vi "Periodic Tasks.vi"(8 "error in":errorcluster) -> ()   [LabVIEW 2018]
doc: "This VI runs in parallel to other tasks. It can contain as many user-defined periodic loops as you need. These can carry out PID or other sorts of timed response."
uses:
  <vilib>/Rock Robotics/WPI/Solenoid/WPI_SolenoidValue.ctl
  <vilib>/Rock Robotics/Network Tables/NT Read Number.vi
  Globals.vi
  <vilib>/Rock Robotics/Network Tables/NT Write String.vi
  <vilib>/Rock Robotics/WPI/Solenoid/WPI_SolenoidSetEnum.vi
  navx-mxp/labview/navX Library v2/navX Library v2.lvlib
panel:
  out "navX axes":T1
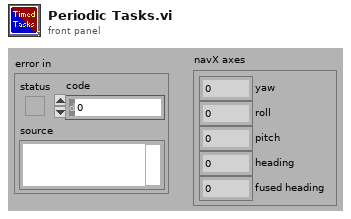
[diagram p1: front panel]
types:
  T1 = cluster{"yaw":dbl, "roll":dbl, "pitch":dbl, "heading":dbl, "fused heading":dbl}
  T2 = typedef "navX Library v2.lvlib/Z900_navX_DeviceTypeDef.ctl" = cluster{"Interface":cluster{"Protocol":T3, "Update Rate (4Hz-100Hz)":u8, "navX Open TypeDef":variant}, "Notify Packet":refnum<notifier>, "Loop VI Refnum":refnum<vi>, "Ready to Close Occurrence Refnum":refnum<k4>}
  T3 = typedef "navX Library v2.lvlib/Z900_navX_ProtocolTypeDef.ctl" = enum16{"SERIAL", "I2C", "SPI"}
  T4 = typedef "WPI_AnalogChannelDevRef.ctl" = cluster{"DevStatus":errorcluster, "Analog Channel":T5}
  T5 = typedef "FPGA_AIChannel.ctl" = enum8{"AI 0", "AI 1", "AI 2", "AI 3", "AI MXP 0", "AI MXP 1", "AI MXP 2", "AI MXP 3", "Invalid"}
  T6 = typedef "WPI_MotorControlDeviceRef.ctl" = cluster{"DeviceStatus":errorcluster, "Type":T7, "PWM":cluster{"PWM Channel":T8, "DeadBand":T9}, "CAN":cluster{"Device Number":u8, "SetOutput VI Ref":variant, "GetOutput VI Ref":variant, "Enable VI Ref":variant, "Disable VI Ref":variant, "Data":variant}, "Invert":bool, "DIO PWM":cluster{"PWM \"Enable\" Channel":T8, "DIOChannel":T10, "PWM Rate":dbl}}
  T7 = typedef "WPI_MotorControlType.ctl" = enum16{"PWM", "CAN", "DIO PWM"}
  T8 = typedef "FPGA_DIOPWMChannel.ctl" = enum8{"PWM 0", "PWM 1", "PWM 2", "PWM 3", "PWM 4", "PWM 5", "PWM 6", "PWM 7", "PWM 8", "PWM 9", "PWM MXP 0", "PWM MXP 1", "PWM MXP 2", "PWM MXP 3", "PWM MXP 4", "PWM MXP 5", "PWM MXP 6", "PWM MXP 7", "PWM MXP 8", "PWM MXP 9", "Invalid"}
  T9 = typedef "WPI_PWMDeadband.ctl" = cluster{"Name":string, "maxPositivePwm":i32, "minPositivePwm":i32, "centerPwm":i32, "maxNegativePwm":i32, "minNegativePwm":i32, "angularRange":u16}
  T10 = typedef "FPGA_DIOChannel.ctl" = enum8{"DIO 0", "DIO 1", "DIO 2", "DIO 3", "DIO 4", "DIO 5", "DIO 6", "DIO 7", "DIO 8", "DIO 9", "DIO MXP 0", "DIO MXP 1", "DIO MXP 2", "DIO MXP 3", "DIO MXP 4", "DIO MXP 5", "DIO MXP 6", "DIO MXP 7", "DIO MXP 8", "DIO MXP 9", "DIO MXP 10", "DIO MXP 11", "DIO MXP 12", "DIO MXP 13", "DIO MXP 14", "DIO MXP 15", "SPI Port CS1", "SPI Port CS2", "SPI Port CS3", "SPI Port MISO", "SPI Port MOSI", "Invalid"}
  T11 = typedef "WPI_EncoderDevRef.ctl" = cluster{"DevStatus":errorcluster, "EncoderIndex":T12, "CounterIndex":T13, "DistancePerCount":dbl, "Decoding Type":T14}
  T12 = typedef "FPGA_EncoderIdx.ctl" = enum8{"Enc 0", "Enc 1", "Enc 2", "Enc 3", "Enc 4", "Enc 5", "Enc 6", "Enc 7", "Invalid"}
  T13 = typedef "FPGA_CounterCtrSystemIndex.ctl" = enum8{"Ctr 0", "Ctr 1", "Ctr 2", "Ctr 3", "Ctr 4", "Ctr 5", "Ctr 6", "Ctr 7", "Invalid"}
  T14 = typedef "WPI_EncoderType.ctl" = enum16{"1x", "2x", "4x"}
  T15 = typedef "WPI_SolenoidDevRef.ctl" = cluster{"DevStatus":errorcluster, "Pneumatics Control Module":u8, "Forward Solenoid Channel":T16, "Reverse Solenoid Channel":T16}
  T16 = typedef "WPI_SolenoidChannel.ctl" = enum8{"Solenoid 0", "Solenoid 1", "Solenoid 2", "Solenoid 3", "Solenoid 4", "Solenoid 5", "Solenoid 6", "Solenoid 7", "Invalid"}
  T17 = typedef "WPI_SolenoidValue.ctl" = enum16{"Off", "On", "Forward", "Reverse"}
  T18 = cluster{"Yaw":dbl, "Roll":dbl, "Pitch":dbl, "Heading":dbl, "Fused Heading":dbl}
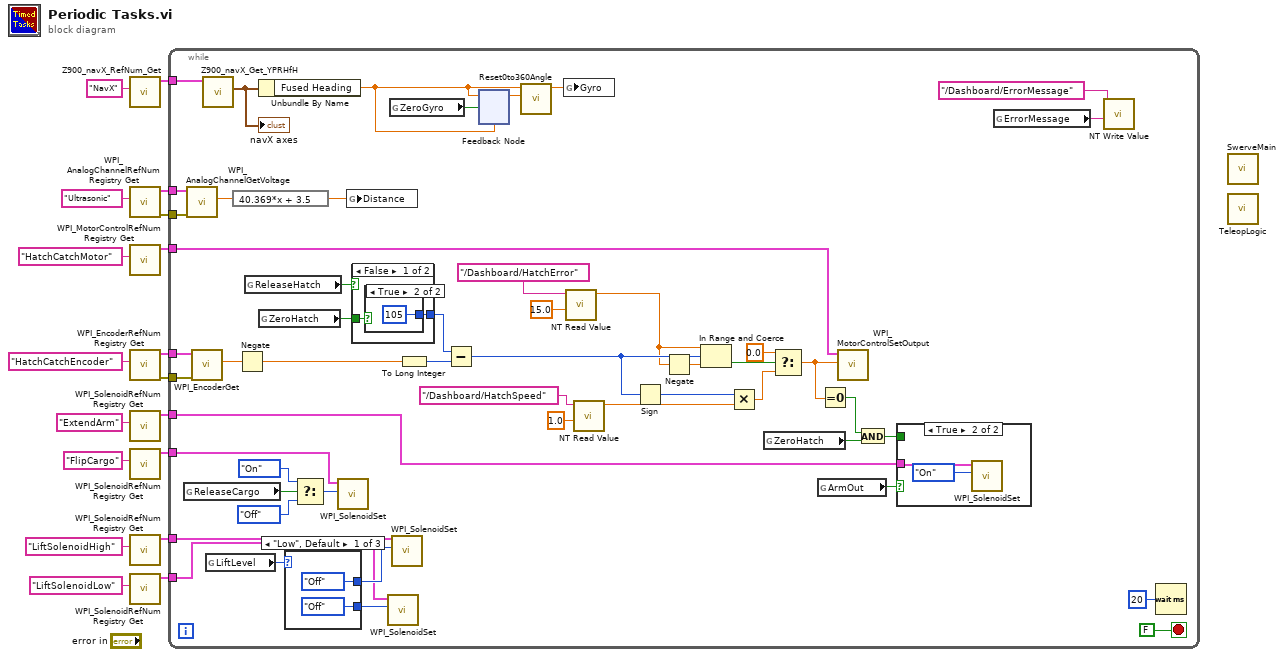
[diagram p0: block diagram]
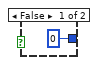
[diagram p3: hidden frame]
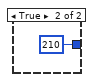
[diagram p4: hidden frame]
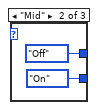
[diagram p5: hidden frame]
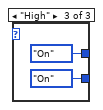
[diagram p6: hidden frame]
diagram:
  n1 = call "Z900_navX_RefNum_Get.vi"("refnum name"="NavX") -> ("navX Device"=w17:T2)  [unwired: 9 in, 1 out]
  n2 = call <vilib>:"WPI_AnalogChannelRefNum Registry Get.vi"("refnum name"="Ultrasonic") -> ("error out"=w15:errorcluster, "AIDeviceRef"=w2:T4)  [unwired: 9 in]
  n3 = call <vilib>:"WPI_MotorControlRefNum Registry Get.vi"("refnum name"="HatchCatchMotor") -> ("MotorControlDevRef"=w14:T6)  [unwired: 9 in, 1 out]
  n4 = call <vilib>:"WPI_EncoderRefNum Registry Get.vi"("refnum name"="HatchCatchEncoder") -> ("error out"=w6:errorcluster, "EncoderDevRef"=w7:T11)  [unwired: 9 in]
  n5 = call <vilib>:"WPI_SolenoidRefNum Registry Get.vi"("refnum name"="ExtendArm") -> ("SolenoidDevRef"=w1:T15)  [unwired: 9 in, 1 out]
  n6 = call <vilib>:"WPI_SolenoidRefNum Registry Get.vi"("refnum name"="FlipCargo") -> ("SolenoidDevRef"=w3:T15)  [unwired: 9 in, 1 out]
  n7 = call <vilib>:"WPI_SolenoidRefNum Registry Get.vi"("refnum name"="LiftSolenoidHigh") -> ("SolenoidDevRef"=w13:T15)  [unwired: 9 in, 1 out]
  n8 = call <vilib>:"WPI_SolenoidRefNum Registry Get.vi"("refnum name"="LiftSolenoidLow") -> ("SolenoidDevRef"=w12:T15)  [unwired: 9 in, 1 out]
  n9 = while {
    tunnel: w17 -> [w42]
    tunnel: w2 -> [w64]
    tunnel: w15 -> [w63]
    tunnel: w14 -> [w33]
    tunnel: w13 -> [w58]
    tunnel: w12 -> [w59]
    tunnel: w7 -> [w57]
    tunnel: w6 -> [w56]
    tunnel: w3 -> [w49]
    tunnel: w1 -> [w21]
    stop <- FALSE stop-if-true
    n10 = global read "Globals.vi" "ReleaseCargo"() -> (w53:bool)
    n11 = call <vilib>:"WPI_AnalogChannelGetVoltage.vi"("error in (no error)"=w63, "AIDeviceRef"=w64) -> ("Voltage"=w32:dbl)  [unwired: 7 in, 2 out]
    n12 = call <vilib>:"WPI_EncoderGet.vi"("error in (no error)"=w56, "EncoderDevRef"=w57) -> ("Distance"=w23:dbl)  [unwired: 4 in, 5 out]
    n13 = call "Z900_navX_Get_YPRHfH.vi"("navX Device"=w42) -> ("YRPHfH"=w67:T18)  [unwired: 7 in, 3 out]
    "navX axes" <- w67
    n14 = global read "Globals.vi" "LiftLevel"() -> (w62:enum16{"Low", "Mid", "High"})
    n15 = expression code="40.369*x + 3.5"(w32) -> (w31:dbl)
    n16 = Negate(x=w23) -> (-x=w22:dbl)
    n17 = global read "Globals.vi" "ReleaseHatch"() -> (w47:bool)
    n18 = Unbundle By Name(w67) -> ("Fused Heading"=w48:dbl)
    n19 = global read "Globals.vi" "ZeroHatch"() -> (w19:bool)
    n20 = case shown="\"Low\", Default" w62 {
      tunnel: [WPI_SolenoidValue."Off" ("Value") WPI_SolenoidValue."Off" ("Value") WPI_SolenoidValue."On" ("Value")] -> w61
      tunnel: [WPI_SolenoidValue."Off" ("Value") WPI_SolenoidValue."On" ("Value") WPI_SolenoidValue."On" ("Value")] -> w60
      frame "Low", Default {
      }
      frame "Mid" {
      }
      frame "High" {
      }
    }
    n21 = Select(t=WPI_SolenoidValue."On" ("Value"), s=w53, f=WPI_SolenoidValue."Off") -> (s? t:f=w50:T17)
    n22 = call-poly <vilib>:"WPI_SolenoidSet.vi"("Value"=w50, "SolenoidDevRef"=w49) -> ()  [unwired: 8 in, 2 out]
    n23 = global write "Globals.vi" "Distance"(w31) -> ()
    n24 = case shown="False" w47 {
      tunnel: w19 -> [w73 _]
      tunnel: [w72 210] -> w24
      frame False {
        n25 = case shown="True" w73 {
          tunnel: [0 105] -> w72
          frame False {
          }
          frame True {
          }
        }
      }
      frame True {
      }
    }
    n26 = call-poly <vilib>:"WPI_SolenoidSet.vi"("Value"=w60, "SolenoidDevRef"=w59) -> ()  [unwired: 8 in, 2 out]
    n27 = global read "Globals.vi" "ZeroGyro"() -> (w65:bool)
    n28 = call-poly <vilib>:"WPI_SolenoidSet.vi"("Value"=w61, "SolenoidDevRef"=w58) -> ()  [unwired: 8 in, 2 out]
    n29 = To Long Integer(number=w22) -> (32bit integer=w46:i32)
    n30 = Subtract(x=w24, y=w46) -> (x-y=w43:i32)
    n31 = feedback-in #1(w48, w65) -> ()
    n32 = feedback #1(w48) -> (w68:dbl)
    n33 = call "Reset0to360Angle.vi"("Offset"=w68, "AngleInput"=w48) -> ("AngleOutput"=w66:dbl)  [unwired: 9 in]
    n34 = global write "Globals.vi" "Gyro"(w66) -> ()
    n35 = call-poly <vilib>:"NT Read Value.vi"("Default Value"=15.0, "Name"="/Dashboard/HatchError") -> ("Numeric"=w25:dbl)  [unwired: 8 in, 1 out]
    n36 = call-poly <vilib>:"NT Read Value.vi"("Default Value"=1.0, "Name"="/Dashboard/HatchSpeed") -> ("Numeric"=w28:dbl)  [unwired: 8 in, 1 out]
    n37 = Sign(1:w43) -> (0:w44:i32)
    n38 = Negate(x=w25) -> (-x=w36:dbl)
    n39 = In Range and Coerce(upper limit=w25, x=w43, lower limit=w36) -> (In Range?=w45:bool)  [unwired: 1 out]
    n40 = Multiply(x=w44, y=w28) -> (x*y=w29:dbl)
    n41 = global read "Globals.vi" "ZeroHatch"() -> (w38:bool)
    n42 = Select(t=0.0, s=w45, f=w29) -> (s? t:f=w40:dbl)
    n43 = global read "Globals.vi" "ArmOut"() -> (w41:bool)
    n44 = Equal To 0?(x=w40) -> (x = 0?=w39:bool)
    n45 = call <vilib>:"WPI_MotorControlSetOutput.vi"("Output"=w40, "MotorControlDevRef"=w33) -> ()  [unwired: 7 in, 3 out]
    n46 = And(x=w39, y=w38) -> (x .and. y?=w37:bool)
    n47 = case shown="True" w41 {
      tunnel: w37 -> [_ _]
      tunnel: w21 -> [_ w71]
      frame False {
      }
      frame True {
        n48 = call-poly <vilib>:"WPI_SolenoidSet.vi"("Value"=WPI_SolenoidValue."On", "SolenoidDevRef"=w71) -> ()  [unwired: 8 in, 2 out]
      }
    }
    n49 = global read "Globals.vi" "ErrorMessage"() -> (w55:string)
    n50 = call-poly <vilib>:"NT Write Value.vi"("String"=w55, "Name"="/Dashboard/ErrorMessage") -> ()  [unwired: 9 in, 1 out]
    n51 = Wait (ms)(milliseconds to wait=u32 20) -> ()  [unwired: 1 out]
  }
  n52 = call "SwerveMain.vi"() -> ()  [unwired: 12 in]
  n53 = call "TeleopLogic.vi"() -> ()  [unwired: 12 in]
